vi "Read Highlighted Row.vi"(8 "error in (no error)":errorcluster, 11 "Scalar MCListbox Refnum":refnum<vi>) -> (0 "error out":errorcluster, 1 "Row Index":i32, 2 "Item Names":string[](array[string]))   [LabVIEW 2020, in "ListboxExtensions.lvlib"]
uses:
  <vilib>/gpm_packages/@cs/listbox/ListboxExtensions.lvlib
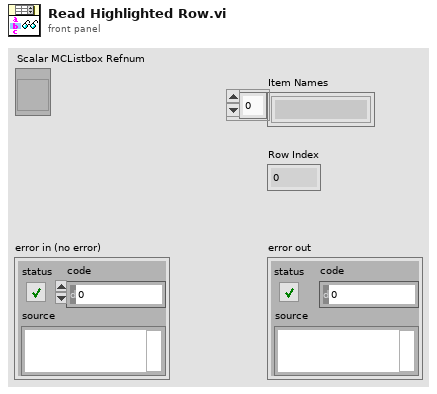
[diagram p1: front panel]
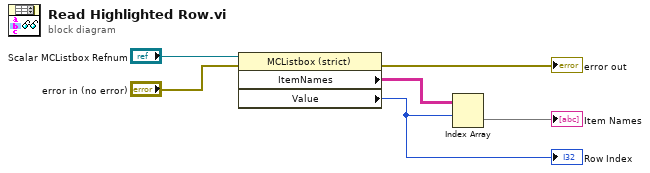
[diagram p0: block diagram]
diagram:
  n1 = property class="MCListbox (strict)"(reference="Scalar MCListbox Refnum", error in="error in (no error)") -> (error out=→"error out":errorcluster, "ItemNames"=w3:string[][], "Value"=w4:i32)  [unwired: 1 out]
  "Row Index" <- w4
  n2 = Index Array(array=w3, index (row)=w4) -> (element=→"Item Names":string[])  [unwired: 1 in]
